vi "NI VeriStand - Get Custom Device Channel Scale Units.vi"(8 "error in (no error)":errorcluster, 11 "Channel Ref in":T1 format="%.0x") -> (0 "error out":errorcluster, 2 "ScaleUnits":string, 3 "Channel Ref out":T1=18446744073709551615 format="%.0x")   [LabVIEW 2020, in "Custom Device API.lvlib"]
uses:
  <vilib>/NI VeriStand/Custom Device API/Custom Device API.lvlib
  <vilib>/NI VeriStand/Custom Device API/Custom Device Item Ref.ctl
  4fe6c354-ac37-4b6d-a87d-92dc250eec85.vi
  <vilib>/NI VeriStand/Custom Device API/Custom Device Offline Path.vi
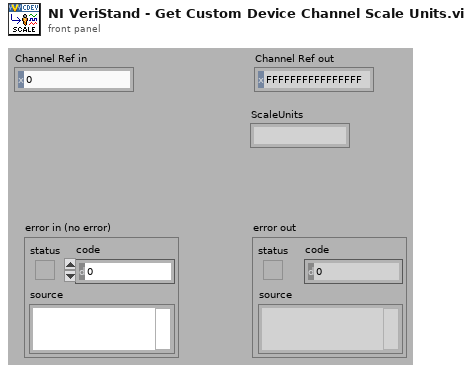
[diagram p1: front panel]
types:
  T1 = typedef "Custom Device API.lvlib/Custom Device Item Ref.ctl" = u64
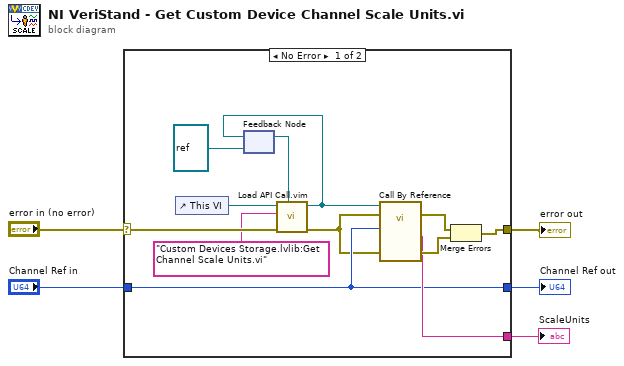
[diagram p0: block diagram]
diagram:
  n1 = case shown="No Error" "error in (no error)" {
    selector: "error in (no error)" -> [w10 w19]
    tunnel: [w16 w19] -> w5
    tunnel: "Channel Ref in" -> [w14 w18]
    tunnel: [w14 w18] -> w3
    tunnel: [w15 _] -> w2
    frame No Error {
      n2 = control-ref of="This VI"() -> (w12:refnum<vi>)
      n3 = feedback #1(refnum<vi> refnum ("type specifier VI Refnum (for type only)")) -> (w13:refnum<vi>)
      n4 = call "Load API Call.vim"("VI reference in"=w13, "error in (no error)"=w10, "VI qualified name"="Custom Devices Storage.lvlib:Get Channel Scale Units.vi", "Caller VI ref"=w12) -> ("error out"=w9:errorcluster, "VI reference"=w8:refnum<vi>)  [unwired: 6 in]
      n5 = feedback-in #1(w8) -> ()
      n6 = call-by-ref "?"(reference=w8, error in=w9, 8:"error in (no error)"=w9, "Channel Ref in"=w14) -> (error out=w6:errorcluster, 0:"error out"=w17:errorcluster, "ScaleUnits"=w15:string)  [unwired: 7 in, 2 out]
      n7 = Merge Errors(w6, w17) -> (w16:errorcluster)
    }
    frame Error {
    }
  }
  "error out" <- w5
  "Channel Ref out" <- w3
  "ScaleUnits" <- w2
